vi "Database Create New Table.vi"(8 "error in (no error)":errorcluster, 9 "column information":T1[](array[typedef]), 10 "table":string, 11 "Database in":refnum<class "DatabaseAPI.lvclass">) -> (0 "error out":errorcluster, 3 "Database out":refnum<class "DatabaseAPI.lvclass">)   [LabVIEW 2015, in "DatabaseAPI.lvclass"]
uses:
  DatabaseAPI.lvclass
  <vilib>/addons/database/Auxilliary.llb/DB Tools Column Info.ctl
  <vilib>/addons/database/Auxilliary.llb/DB Tools DataTypes.ctl
  DatabaseAPI.lvclass/DatabaseAPI.ctl
  <vilib>/addons/database/Connection.llb/DB Tools Open Connec (String).vi
  <vilib>/addons/database/NI_Database_API.lvlib
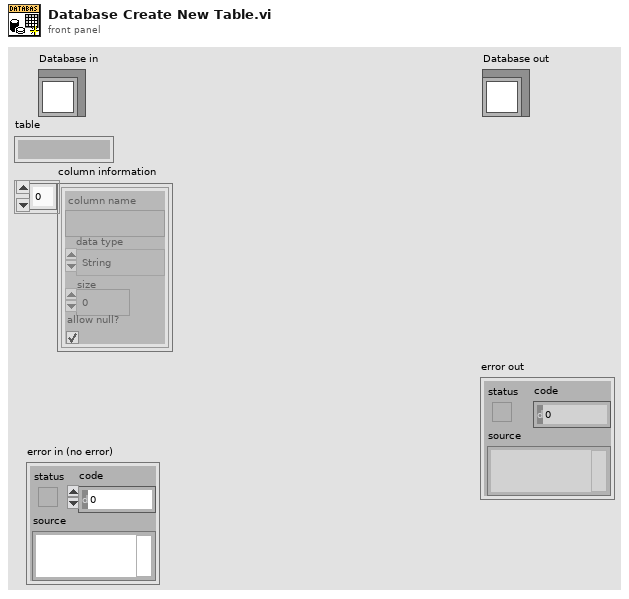
[diagram p1: front panel]
types:
  T1 = typedef "NI_Database_API.lvlib/DB Tools Column Info.ctl" = cluster{"column name":string, "data type":T2, "size":i32, "allow null?":bool}
  T2 = typedef "NI_Database_API.lvlib/DB Tools DataTypes.ctl" = enum16{"String", "Long (I32)", "Single (SGL)", "Double (DBL)", "Date/Time", "Binary"}
  T3 = typedef "NI_Database_API.lvlib/Conn ObjectReference.ctl" = refnum<k1>
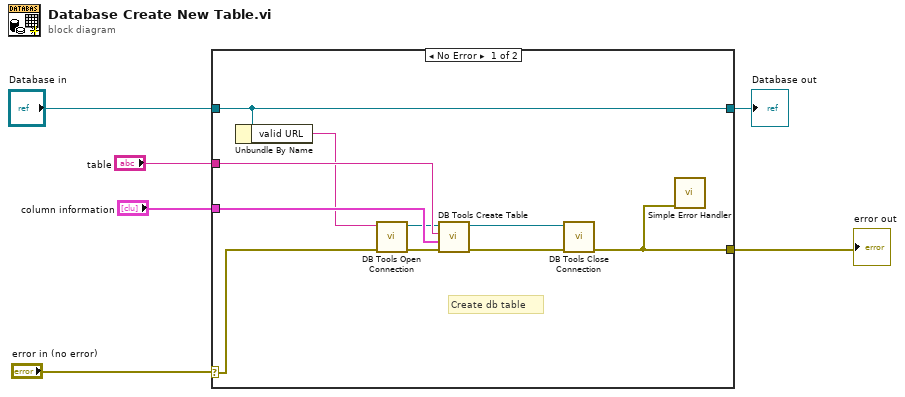
[diagram p0: block diagram]
diagram:
  n1 = case shown="No Error" "error in (no error)" {
    selector: "error in (no error)" -> [w14 w18]
    tunnel: [w10 w18] -> w1
    tunnel: [w8 w17] -> w5
    tunnel: "Database in" -> [w8 w17]
    tunnel: "table" -> [w16 _]
    tunnel: "column information" -> [w15 _]
    frame No Error {
      # "Create db table"
      n2 = Unbundle By Name(w8) -> ("valid URL"=w7:string)
      n3 = call-poly <vilib>:"DB Tools Open Connection.vi"("error in (no error)"=w14, "connection information"=w7) -> ("error out"=w9:errorcluster, "connection reference"=w13:T3)  [unwired: 6 in]
      n4 = call <vilib>:"DB Tools Create Table.vi"("error in (no error)"=w9, "column information"=w15, "table"=w16, "connection reference"=w13) -> ("error out"=w11:errorcluster, "connection reference out"=w12:T3)  [unwired: 4 in]
      n5 = call <vilib>:"DB Tools Close Connection.vi"("error in (no error)"=w11, "connection reference"=w12) -> ("error out"=w10:errorcluster)  [unwired: 5 in]
      n6 = call <vilib>:"Simple Error Handler.vi"("error in (no error)"=w10) -> ()  [unwired: 4 in, 5 out]
    }
    frame Error {
    }
  }
  "error out" <- w1
  "Database out" <- w5
